vi "NET SetInput.vi"(4 "Mean":dbl[](array[numeric]), 6 "Scalefactor":dbl=1.0, 8 "error in (no error)":errorcluster, 9 "Name":string, 10 "Blob":refnum<class "Blob.lvclass">, 11 "NET in":refnum<class "NET.lvclass">) -> (0 "error out":errorcluster, 2 "Blob out":refnum<class "Blob.lvclass">, 3 "NET out":refnum<class "NET.lvclass">)   [LabVIEW 2020, in "OpenLvVision_OpenCv.lvlib" / "NET.lvclass"]
doc: "Sets the new input value for the network."
uses:
  NET.lvclass
  C:/Users/lukas/Downloads/OpenLvVision_OpenCv/SourceCode/LabView/OpenLvVision_OpenCv/_LvHelpers/EdvrObject/EdvrObject.lvclass
  Blob/Blob.lvclass
  _LvHelpers/EdvrObject/EdvrObject.lvclass/EdvrObject.ctl
  OpenLvVision_OpenCv.lvlib
  _LvHelpers/EdvrObject/EdvrObject.lvclass
  Dlls/OlvOpenCvWrapper.dll
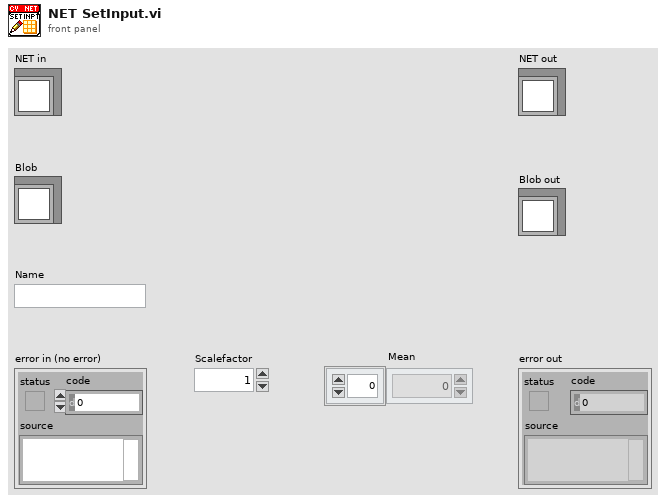
[diagram p1: front panel]
types:
  T1 = typedef "OpenLvVision_OpenCv.lvlib/EdvrObject.lvclass/Edvr.ctl" = refnum<data-value>
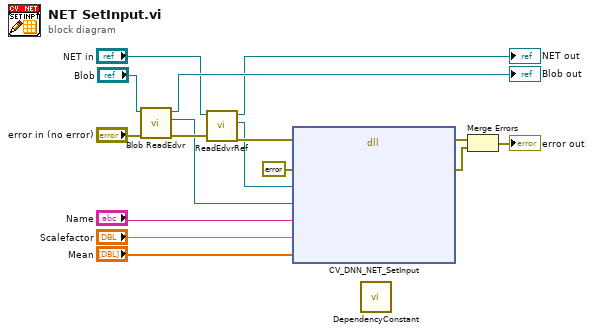
[diagram p0: block diagram]
diagram:
  n1 = call "Blob ReadEdvr.vi"("error in (no error)"="error in (no error)", "Blob in"="Blob") -> ("error out"=w8:errorcluster, "Edvr"=w7:T1, "Blob out"=→"Blob out":refnum<class "Blob.lvclass">)  [unwired: 7 in]
  n2 = call "ReadEdvrRef.vi"("error in (no error)"=w8, "EdvrObject in"="NET in") -> ("error out"=w12:errorcluster, "Edvr"=w11:T1, "EdvrObject out"=→"NET out":refnum<class "NET.lvclass">)  [unwired: 7 in]
  n3 = dll-call lib="C:/Users/lukas/Downloads/OpenLvVision_OpenCv/SourceCode/LabView/OpenLvVision_OpenCv/Dlls/OlvOpenCvWrapper.dll" fn="CV_DNN_NET_SetInput"(error in=w12, "Error"=errorcluster {"status"=FALSE, "code"=0, "source"=""} ("error out"), "edvrRef"=w11, "edvrRefBlob"=w7, "ouptuName"="Name", "scalefactor"="Scalefactor", "mean"="Mean") -> (error out=w15:errorcluster, "Error"=w14:errorcluster)  [unwired: 8 in, 1 out]
  n4 = call "DependencyConstant.vi"() -> ()  [unwired: 12 in]
  n5 = Merge Errors(w15, w14) -> (→"error out":errorcluster)
